vi "ex_2.vi"(7 "Reset (T)/Count (F)":bool=TRUE, 8 "error in (no error)":errorcluster) -> (0 "error out":errorcluster, 3 "Counter":i32)   [LabVIEW 2020]
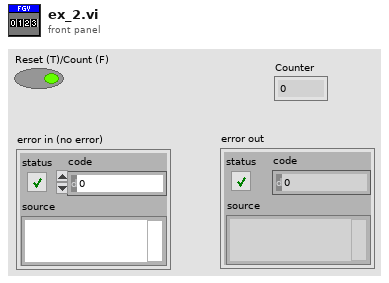
[diagram p1: front panel]
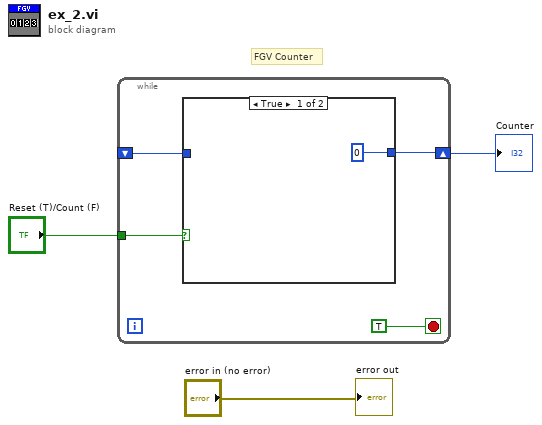
[diagram p0: block diagram]
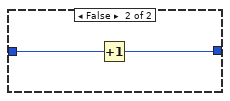
[diagram p2: hidden frame]
diagram:
  # "FGV Counter"
  n1 = while {
    shift-right: [w6] -> w3
    shift-left: _ -> [w5]
    tunnel: "Reset (T)/Count (F)" -> [w4]
    stop <- TRUE stop-if-true
    n2 = case shown="True" w4 {
      tunnel: [0 w9] -> w6
      tunnel: w5 -> [_ w10]
      frame True {
      }
      frame False {
        n3 = Increment(x=w10) -> (x+1=w9:i32)
      }
    }
  }
  "Counter" <- w3
  "error out" <- "error in (no error)"
